vi "integrate_resonance_flexRIO.vi"(5 "waiting iterations per pixel":u32, 7 "integration iterations per pixel":u32, 9 "iteration counter in":u32, 10 "sampling values in":T1, 11 "integration cluster in":T2) -> (1 "finished?":bool, 2 "iteration counter out":u32, 3 "integration cluster out":T2)   [LabVIEW 2010]
uses:
  integration_cluster_flexRIO.ctl
  channels_cluster_flexRIO.ctl
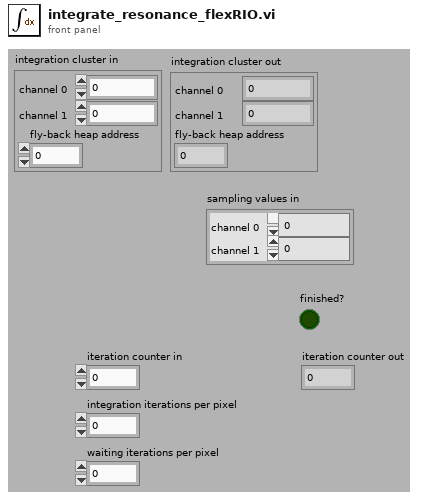
[diagram p1: front panel]
types:
  T1 = typedef "channels_cluster_flexRIO.ctl" = cluster{"channel 0":u32, "channel 1":u32}
  T2 = typedef "integration_cluster_flexRIO.ctl" = cluster{"channel 0":u32, "channel 1":u32, "fly-back heap address":u32}
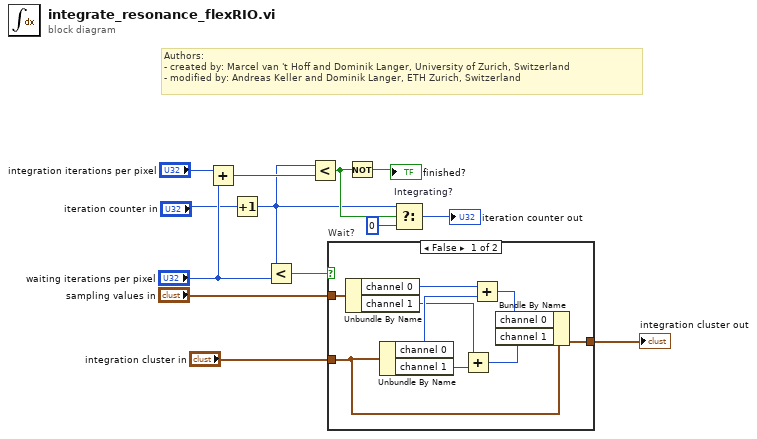
[diagram p0: block diagram]
diagram:
  # "Authors: \n- created by: Marcel van 't Hoff and Dominik Langer, University of Zurich, Switzerland\n- modified by: Andreas Keller and Dominik Langer, ETH Zurich, Switzerland"
  n1 = Add(x="integration iterations per pixel", y="waiting iterations per pixel") -> (x+y=w9:u32)
  n2 = Increment(x="iteration counter in") -> (x+1=w6:u32)
  n3 = Less?(x=w6, y="waiting iterations per pixel") -> (x < y?=w10:bool)
  n4 = Less?(x=w6, y=w9) -> (x < y?=w7:bool)
  n5 = case "Wait?" shown="False" w10 {
    tunnel: "sampling values in" -> [w18 _]
    tunnel: "integration cluster in" -> [w17 w23]
    tunnel: [w14 w23] -> w2
    frame False {
      n6 = Unbundle By Name(w18) -> ("channel 0"=w22:u32, "channel 1"=w20:u32)
      n7 = Unbundle By Name(w17) -> ("channel 0"=w21:u32, "channel 1"=w19:u32)
      n8 = Add(x=w20, y=w19) -> (x+y=w15:u32)
      n9 = Add(x=w22, y=w21) -> (x+y=w16:u32)
      n10 = Bundle By Name(cluster=w17, "channel 0"=w16, "channel 1"=w15) -> (w14:T2)
    }
    frame True {
    }
  }
  "integration cluster out" <- w2
  n11 = Not(x=w7) -> (.not. x?=→"finished?":bool)
  n12 = Select "Integrating?"(t=w6, s=w7, f=u32 0) -> (s? t:f=→"iteration counter out":u32)
